vi "test.vi"() -> ()   [LabVIEW 2016]
uses:
  <vilib>/ptbypt/NI_PtbyPt.lvlib
panel:
  in  "配置信息":cluster{"周期模式":T1, "定点周期":T2, "间隔启动":T4} {"定点周期"."启动命令 24" items=["", "水样测试", "标样核查", "零点核查", "跨度核查", "空白测试", "平行样测试", "加标回收", "空白校准", "标样校准"]; "定点周期"."启动命令 23" items=["", "水样测试", "标样核查", "零点核查", "跨度核查", "空白测试", "平行样测试", "加标回收", "空白校准", "标样校准"]; "定点周期"."启动命令 22" items=["", "水样测试", "标样核查", "零点核查", "跨度核查", "空白测试", "平行样测试", "加标回收", "空白校准", "标样校准"]; "定点周期"."启动命令 21" items=["", "水样测试", "标样核查", "零点核查", "跨度核查", "空白测试", "平行样测试", "加标回收", "空白校准", "标样校准"]; "定点周期"."启动命令 20" items=["", "水样测试", "标样核查", "零点核查", "跨度核查", "空白测试", "平行样测试", "加标回收", "空白校准", "标样校准"]; "定点周期"."启动命令 19" items=["", "水样测试", "标样核查", "零点核查", "跨度核查", "空白测试", "平行样测试", "加标回收", "空白校准", "标样校准"]; "定点周期"."启动命令 18" items=["", "水样测试", "标样核查", "零点核查", "跨度核查", "空白测试", "平行样测试", "加标回收", "空白校准", "标样校准"]; "定点周期"."启动命令 17" items=["", "水样测试", "标样核查", "零点核查", "跨度核查", "空白测试", "平行样测试", "加标回收", "空白校准", "标样校准"]; "定点周期"."启动命令 16" items=["", "水样测试", "标样核查", "零点核查", "跨度核查", "空白测试", "平行样测试", "加标回收", "空白校准", "标样校准"]; "定点周期"."启动命令 15" items=["", "水样测试", "标样核查", "零点核查", "跨度核查", "空白测试", "平行样测试", "加标回收", "空白校准", "标样校准"]; "定点周期"."启动命令 14" items=["", "水样测试", "标样核查", "零点核查", "跨度核查", "空白测试", "平行样测试", "加标回收", "空白校准", "标样校准"]; "定点周期"."启动命令 13" items=["", "水样测试", "标样核查", "零点核查", "跨度核查", "空白测试", "平行样测试", "加标回收", "空白校准", "标样校准"]; "定点周期"."启动命令 12" items=["", "水样测试", "标样核查", "零点核查", "跨度核查", "空白测试", "平行样测试", "加标回收", "空白校准", "标样校准"]; "定点周期"."启动命令 11" items=["", "水样测试", "标样核查", "零点核查", "跨度核查", "空白测试", "平行样测试", "加标回收", "空白校准", "标样校准"]; "定点周期"."启动命令 10" items=["", "水样测试", "标样核查", "零点核查", "跨度核查", "空白测试", "平行样测试", "加标回收", "空白校准", "标样校准"]; "定点周期"."启动命令 9" items=["", "水样测试", "标样核查", "零点核查", "跨度核查", "空白测试", "平行样测试", "加标回收", "空白校准", "标样校准"]; "定点周期"."启动命令 8" items=["", "水样测试", "标样核查", "零点核查", "跨度核查", "空白测试", "平行样测试", "加标回收", "空白校准", "标样校准"]; "定点周期"."启动命令 7" items=["", "水样测试", "标样核查", "零点核查", "跨度核查", "空白测试", "平行样测试", "加标回收", "空白校准", "标样校准"]; "定点周期"."启动命令 6" items=["", "水样测试", "标样核查", "零点核查", "跨度核查", "空白测试", "平行样测试", "加标回收", "空白校准", "标样校准"]; "定点周期"."启动命令 5" items=["", "水样测试", "标样核查", "零点核查", "跨度核查", "空白测试", "平行样测试", "加标回收", "空白校准", "标样校准"]; "定点周期"."启动命令 4" items=["", "水样测试", "标样核查", "零点核查", "跨度核查", "空白测试", "平行样测试", "加标回收", "空白校准", "标样校准"]; "定点周期"."启动命令 3" items=["", "水样测试", "标样核查", "零点核查", "跨度核查", "空白测试", "平行样测试", "加标回收", "空白校准", "标样校准"]; "定点周期"."启动命令 2" items=["", "水样测试", "标样核查", "零点核查", "跨度核查", "空白测试", "平行样测试", "加标回收", "空白校准", "标样校准"]; "定点周期"."启动命令" items=["", "水样测试", "标样核查", "零点核查", "跨度核查", "空白测试", "平行样测试", "加标回收", "空白校准", "标样校准"]; "间隔启动"."启动命令" items=["", "水样测试", "标样核查", "零点核查", "跨度核查", "空白测试", "平行样测试", "加标回收", "空白校准", "标样校准"]}
  out "周期设置 2":cluster{"启动":bool, "控制命令":T5}
  out "数值":i32
  out "间隔计时":dbl
  out "启动次数":i32
  out "仪器运行状态":bool
  out "最近一次结束时间":timestamp
  out "最近一次启动时间":timestamp
  in  "周期设置":cluster{"启动":bool, "控制命令":T5}(xcontrol)
  in  "仪器运行状态 2":bool
  out "数组":T6(array[cluster])
  # "分钟"
  # "次"
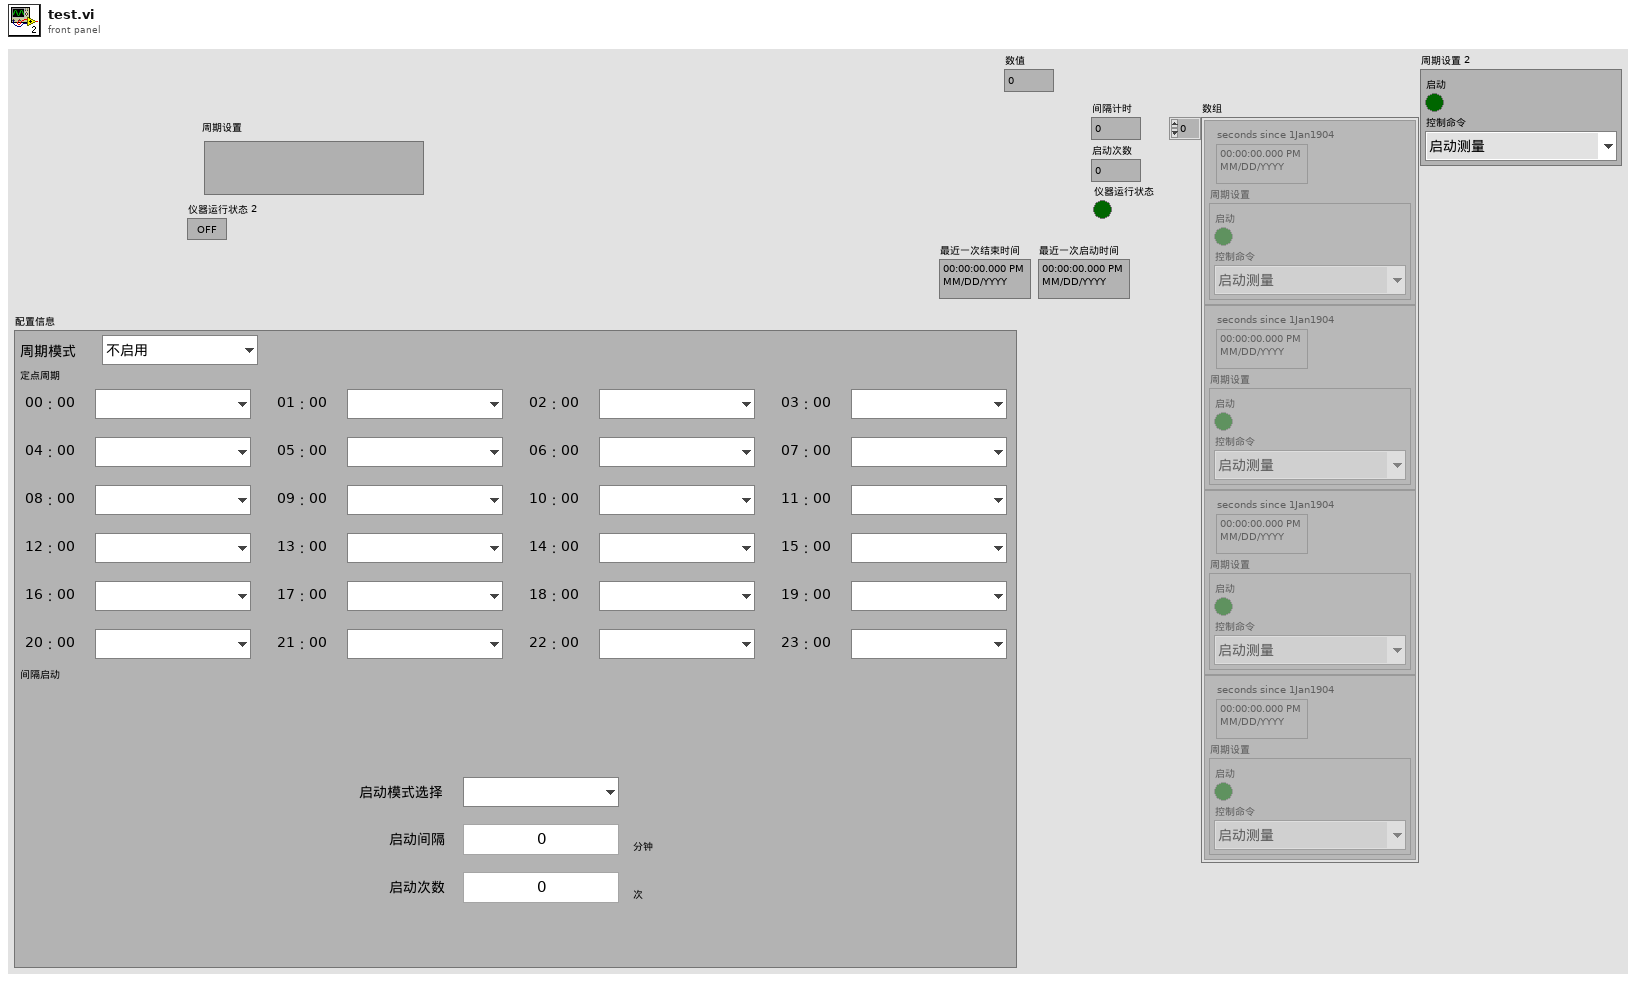
[diagram p1: front panel]
types:
  T1 = typedef "定时设置.xctl/周期模式设置.ctl" = enum16{"不启用", "定点模式", "间隔模式"}
  T2 = typedef "定时设置.xctl/定点周期设置.ctl" = cluster{"启动命令":T3, "启动命令 2":T3, "启动命令 3":T3, "启动命令 4":T3, "启动命令 5":T3, "启动命令 6":T3, "启动命令 7":T3, "启动命令 8":T3, "启动命令 9":T3, "启动命令 10":T3, "启动命令 11":T3, "启动命令 12":T3, "启动命令 13":T3, "启动命令 14":T3, "启动命令 15":T3, "启动命令 16":T3, "启动命令 17":T3, "启动命令 18":T3, "启动命令 19":T3, "启动命令 20":T3, "启动命令 21":T3, "启动命令 22":T3, "启动命令 23":T3, "启动命令 24":T3}
  T3 = typedef "定时设置.xctl/启动命令选择.ctl" = u16
  T4 = typedef "定时设置.xctl/间隔启动设置.ctl" = cluster{"启动命令":T3, "启动间隔":dbl, "启动次数":i32}
  T5 = typedef "定时设置.xctl/国标控制命令.ctl" = enum16{"启动测量", "标样核查", "零点核查", "跨度核查", "空白测试", "平行样测试", "加标回收", "空白校准", "标样校准", "初始化（清洗）", "停止测试", "仪器重启", "校时", "模式设置", "测量间隔设置"}
  T6 = cluster{"seconds since 1Jan1904":timestamp, "周期设置":cluster{"启动":bool, "控制命令":T5}}[]
  T7 = cluster{"seconds since 1Jan1904":timestamp, "周期设置":cluster{"启动":bool, "控制命令":T5}}
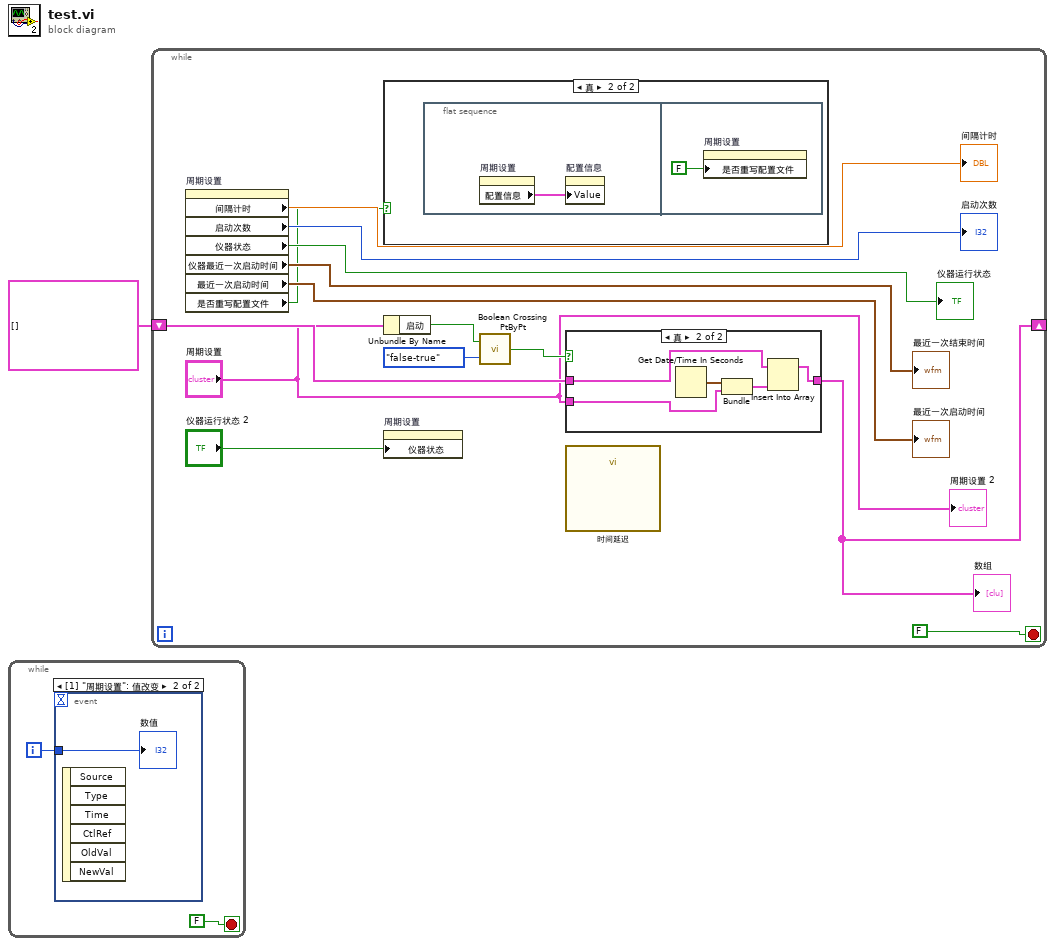
[diagram p0: block diagram]
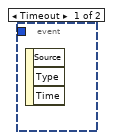
[diagram p2: hidden frame]
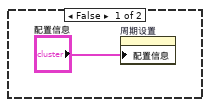
[diagram p3: hidden frame]
diagram:
  n1 = while {
    i -> [w2]
    stop <- FALSE stop-if-true
    n2 = event shown="[1] \"周期设置\": 值改变" {
      selector: _ -> [_ _]
      dyn-events: _ -> [_ _]
      timeout: _ -> [_ _]
      tunnel: w2 -> [_ w4]
      event Timeout {
        n3 = event-data() -> ()  [unwired: 1 in, 3 out]
      }
      event "周期设置": Value Change {
        n4 = event-data() -> ()  [unwired: 1 in, 6 out]
        "数值" <- w4
      }
    }
  }
  n5 = while {
    shift-right: [w9] -> _
    shift-left: T6 [] -> [w8]
    stop <- FALSE stop-if-true
    n6 = property on="周期设置" class="定时设置 (严格)"() -> ("间隔计时"=→"间隔计时":dbl, "启动次数"=→"启动次数":i32, "仪器状态"=→"仪器运行状态":bool, "仪器最近一次启动时间"=→"最近一次结束时间":timestamp, "最近一次启动时间"=→"最近一次启动时间":timestamp, "是否重写配置文件"=w6:bool)  [unwired: 2 in, 2 out]
    n7 = case shown="真" w6 {
      frame False {
        n8 = property on="周期设置" class="定时设置 (严格)"("配置信息"="配置信息") -> ()  [unwired: 2 in, 2 out]
      }
      frame True {
        n9 = flat-sequence {
          frame #0 {
            n10 = property on="周期设置" class="定时设置 (严格)"() -> ("配置信息"=w20:cluster{"周期模式":T1, "定点周期":T2, "间隔启动":T4})  [unwired: 2 in, 2 out]
            n11 = property on="配置信息" class="Clust (严格)"("Value"=w20) -> ()  [unwired: 2 in, 2 out]
          }
          frame #1 {
            n12 = property on="周期设置" class="定时设置 (严格)"("是否重写配置文件"=FALSE) -> ()  [unwired: 2 in, 2 out]
          }
        }
      }
    }
    n13 = Unbundle By Name("周期设置") -> ("启动"=w12:bool)
    n14 = property on="周期设置" class="定时设置 (严格)"("仪器状态"="仪器运行状态 2") -> ()  [unwired: 2 in, 2 out]
    n15 = call <vilib>:"Boolean Crossing PtByPt.vi"("direction"=enum16{"either", "false-true", "true-false"}."false-true", "input"=w12) -> ("crossing"=w10:bool)  [unwired: 1 in]
    n16 = case shown="真" w10 {
      tunnel: "周期设置" -> [_ w26]
      tunnel: [w22 w24] -> w9
      tunnel: w8 -> [w22 w23]
      frame False {
      }
      frame True {
        n17 = Get Date/Time In Seconds() -> (seconds since 1Jan1904=w27:timestamp)
        n18 = Bundle("seconds since 1Jan1904"=w27, "周期设置"=w26) -> (w25:T7)  [unwired: 1 in]
        n19 = Insert Into Array(array=w23, new element=w25) -> (w24:T6)  [unwired: 1 in]
      }
    }
    "数组" <- w9
    n20 = call "时间延迟"() -> ()  [unwired: 11 in, 1 out]
    "周期设置 2" <- "周期设置"
  }
